vi "benchmark-memory.vi"(11 "iterations":i32=1000000) -> (0 "mean (s)":dbl format="%#_6f", 1 "max value":dbl format="%#_6f", 2 "min value (s)":dbl format="%#_6f", 3 "data":dbl[][](array[numeric]), 6 "duration (s)":dbl)   [LabVIEW 2020]
uses:
  <vilib>/numeric/Random Number (Range) DBL.vi
  <vilib>/Analysis/baseanly.llb/Mean (DBL).vi
  <vilib>/Analysis/NI_AALBase.lvlib
panel:
  out "loop delay":dbl[][](graph)
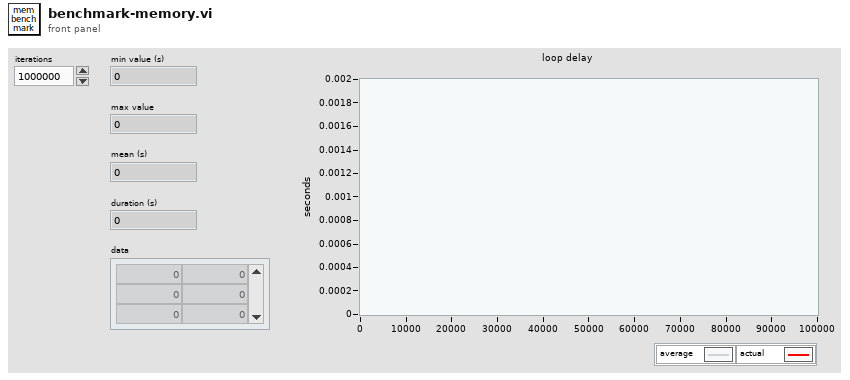
[diagram p1: front panel]
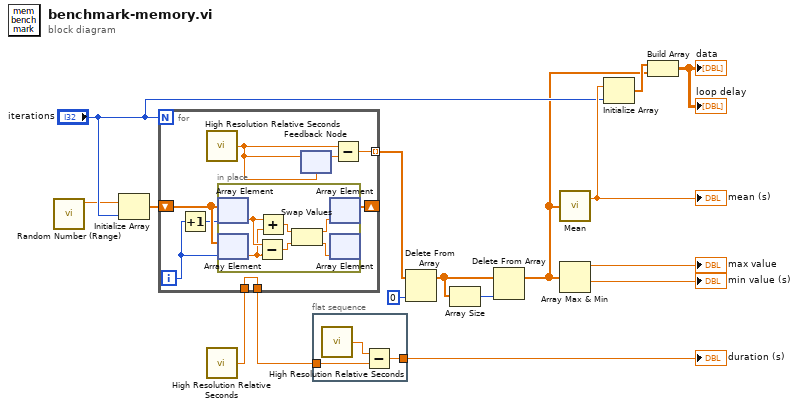
[diagram p0: block diagram]
diagram:
  n1 = call-poly <vilib>:"Random Number (Range).vi"() -> ("number"=w6:dbl)  [unwired: 11 in]
  n2 = Initialize Array(w6, "iterations") -> (w5:dbl[])
  n3 = call <vilib>:"High Resolution Relative Seconds.vi"() -> ("relative seconds"=w10:dbl)
  n4 = for {
    N: "iterations" -> [_]
    tunnel: [w23] -> w14 mode=indexing
    shift-right: [w20] -> _
    shift-left: w5 -> [w19]
    tunnel: w10 -> [w21]
    tunnel: [w21] -> w9
    i -> [w17]
    n5 = Increment(x=w17) -> (x+1=w18:i32)
    n6 = call <vilib>:"High Resolution Relative Seconds.vi"() -> ("relative seconds"=w22:dbl)
    n7 = in-place {
      n8 = in-place-array #1(w19, w18) -> (w27:dbl)
      n9 = in-place-array #2(w19, w17) -> (w26:dbl)
      n10 = Subtract(x=w27, y=w26) -> (x-y=w28:dbl)
      n11 = Add(x=w27, y=w26) -> (x+y=w25:dbl)
      n12 = Swap Values(12:w25, 14:w28) -> (1:w30:dbl, 3:w29:dbl)  [unwired: 1 in]
      n13 = in-place-array #1(w30) -> (w20:dbl[])  [unwired: 1 out]
      n14 = in-place-array #2(w29) -> ()  [unwired: 2 out]
    }
    n15 = feedback-in #3(w22) -> ()
    n16 = feedback #3(w22) -> (w24:dbl)
    n17 = Subtract(x=w22, y=w24) -> (x-y=w23:dbl)
  }
  n18 = flat-sequence {
    tunnel: w9 -> [w32]
    tunnel: [w31] -> w8
    frame #0 {
      n19 = call <vilib>:"High Resolution Relative Seconds.vi"() -> ("relative seconds"=w33:dbl)
      n20 = Subtract(x=w33, y=w32) -> (x-y=w31:dbl)
    }
  }
  n21 = Delete From Array(array=w14, index=0) -> (array with subset deleted=w1:dbl[])  [unwired: 1 in, 1 out]
  n22 = Array Size(array=w1) -> (size(s)=w2:i32)
  n23 = Delete From Array(array=w1, index=w2) -> (array with subset deleted=w3:dbl[])  [unwired: 1 in, 1 out]
  n24 = call-poly <vilib>:"Mean.vi"("X"=w3) -> ("mean"=w12:dbl)  [unwired: 1 out]
  "mean (s)" <- w12
  n25 = Array Max & Min(array=w3) -> (max value=→"max value":dbl, min value=→"min value (s)":dbl)  [unwired: 2 out]
  n26 = Initialize Array(w12, "iterations") -> (w11:dbl[])
  n27 = Build Array(w11, w3) -> (→"data" →"loop delay":dbl[][])
  "duration (s)" <- w8
